vi "MAIN.vi"() -> (2 "digitale waarden reflectiesensor":i32[](array[numeric]))   [LabVIEW 2019]
uses:
  <vilib>/myRIO/Common/Instrument Driver Framework/Utilities/typedefs/Analog Scaling Constants.ctl
  <vilib>/myRIO/Common/Instrument Driver Framework/Utilities/typedefs/Analog Scaling Constants List.ctl
  <vilib>/myRIO/Common/Instrument Driver Framework/myRIO v1.0/AO/typedefs/AO Channels Enum.ctl
  <vilib>/myRIO/Common/Instrument Driver Framework/myRIO v1.0/AO/typedefs/AO Channels List.ctl
  <vilib>/myRIO/Common/Instrument Driver Framework/Utilities/typedefs/Generic FPGA Reference.ctl
  <vilib>/myRIO/Common/Instrument Driver Framework/Utilities/typedefs/myRIO v1.0 Reference.ctl
  <vilib>/myRIO/Common/Instrument Driver Framework/Utilities/typedefs/Hardware Version Enum.ctl
  <vilib>/myRIO/Common/Instrument Driver Framework/Utilities/typedefs/myRIO Generic Hardware Reference.ctl
  <vilib>/myRIO/Instrument Drivers/Onboard IO/AO/typedefs/AO Reference.ctl
  <vilib>/myRIO/Instrument Drivers/Onboard IO/AO/AO.lvlib
  <vilib>/myRIO/Instrument Drivers/Onboard IO/AO/vis/Write.vi
  <vilib>/userDefined/High Color/nirio_resource_hc.ctl
  <vilib>/myRIO/Common/Instrument Driver Framework/myRIO v1.0/AO/vis/myRIO v1.1 Open AO.vi
  <vilib>/myRIO/Instrument Drivers/Onboard IO/AO/vis/myRIO AO Open.xnode
  <vilib>/myRIO/Common/Instrument Driver Framework/Utilities/vis/Is FPGA Ref Available.vi
  <vilib>/myRIO/Express VI/Onboard IO/AO/AO Express VI.xnode
  <vilib>/myRIO/Common/Instrument Driver Framework/myRIO v1.0/AI/typedefs/AI Channels Enum.ctl
  <vilib>/myRIO/Common/Instrument Driver Framework/myRIO v1.0/AI/typedefs/AI Channels List.ctl
  <vilib>/myRIO/Instrument Drivers/Onboard IO/AI/typedefs/AI Reference.ctl
  <vilib>/myRIO/Instrument Drivers/Onboard IO/AI/AI.lvlib
  <vilib>/myRIO/Instrument Drivers/Onboard IO/AI/vis/Read.vi
  <vilib>/myRIO/Common/Instrument Driver Framework/myRIO v1.0/AI/vis/myRIO v1.1 Open AI.vi
  <vilib>/myRIO/Instrument Drivers/Onboard IO/AI/vis/myRIO AI Open.xnode
  <vilib>/myRIO/Express VI/Onboard IO/AI/AI Express VI.xnode
  <vilib>/myRIO/Express VI/Onboard IO/DI/DI Express VI.xnode
  <vilib>/myRIO/Instrument Drivers/Onboard IO/DIO/vis/Read.vi
  <vilib>/myRIO/Instrument Drivers/Onboard IO/DIO/DIO.lvlib
  <vilib>/myRIO/Common/Instrument Driver Framework/myRIO v1.0/DIO/typedefs/DIO Channels Enum.ctl
  <vilib>/myRIO/Common/Instrument Driver Framework/myRIO v1.0/DIO/typedefs/DIO Channels List.ctl
  <vilib>/myRIO/Instrument Drivers/Onboard IO/DIO/typedefs/DIO Reference.ctl
  <vilib>/myRIO/Instrument Drivers/Onboard IO/DIO/vis/myRIO DIO Open.xnode
  <vilib>/myRIO/Common/Instrument Driver Framework/myRIO v1.0/DIO/vis/myRIO v1.1 Open DIO.vi
panel:
  in  "stoppen":bool
  in  "rechts draaien achteruit":bool
  in  "links draaien achteruit":bool
  in  "snelheid":dbl
  in  "rechts draaien":bool
  in  "links draaien":bool
  in  "achterwaarts":bool
  in  "voorwaarts":bool
  out "boolean afstandssensor":bool
  out "High 2":u8[](array[numeric])
  out "Low 2":u8[](array[numeric])
  out "error out":errorcluster
  in  "error in (no error)":errorcluster
  out "Total":u32
  in  "Low":string="–"
  in  "High":string="—"
  out "analoge waarden refelectiesensor":dbl[](array[numeric])
  in  "manuele bedieningknop":bool
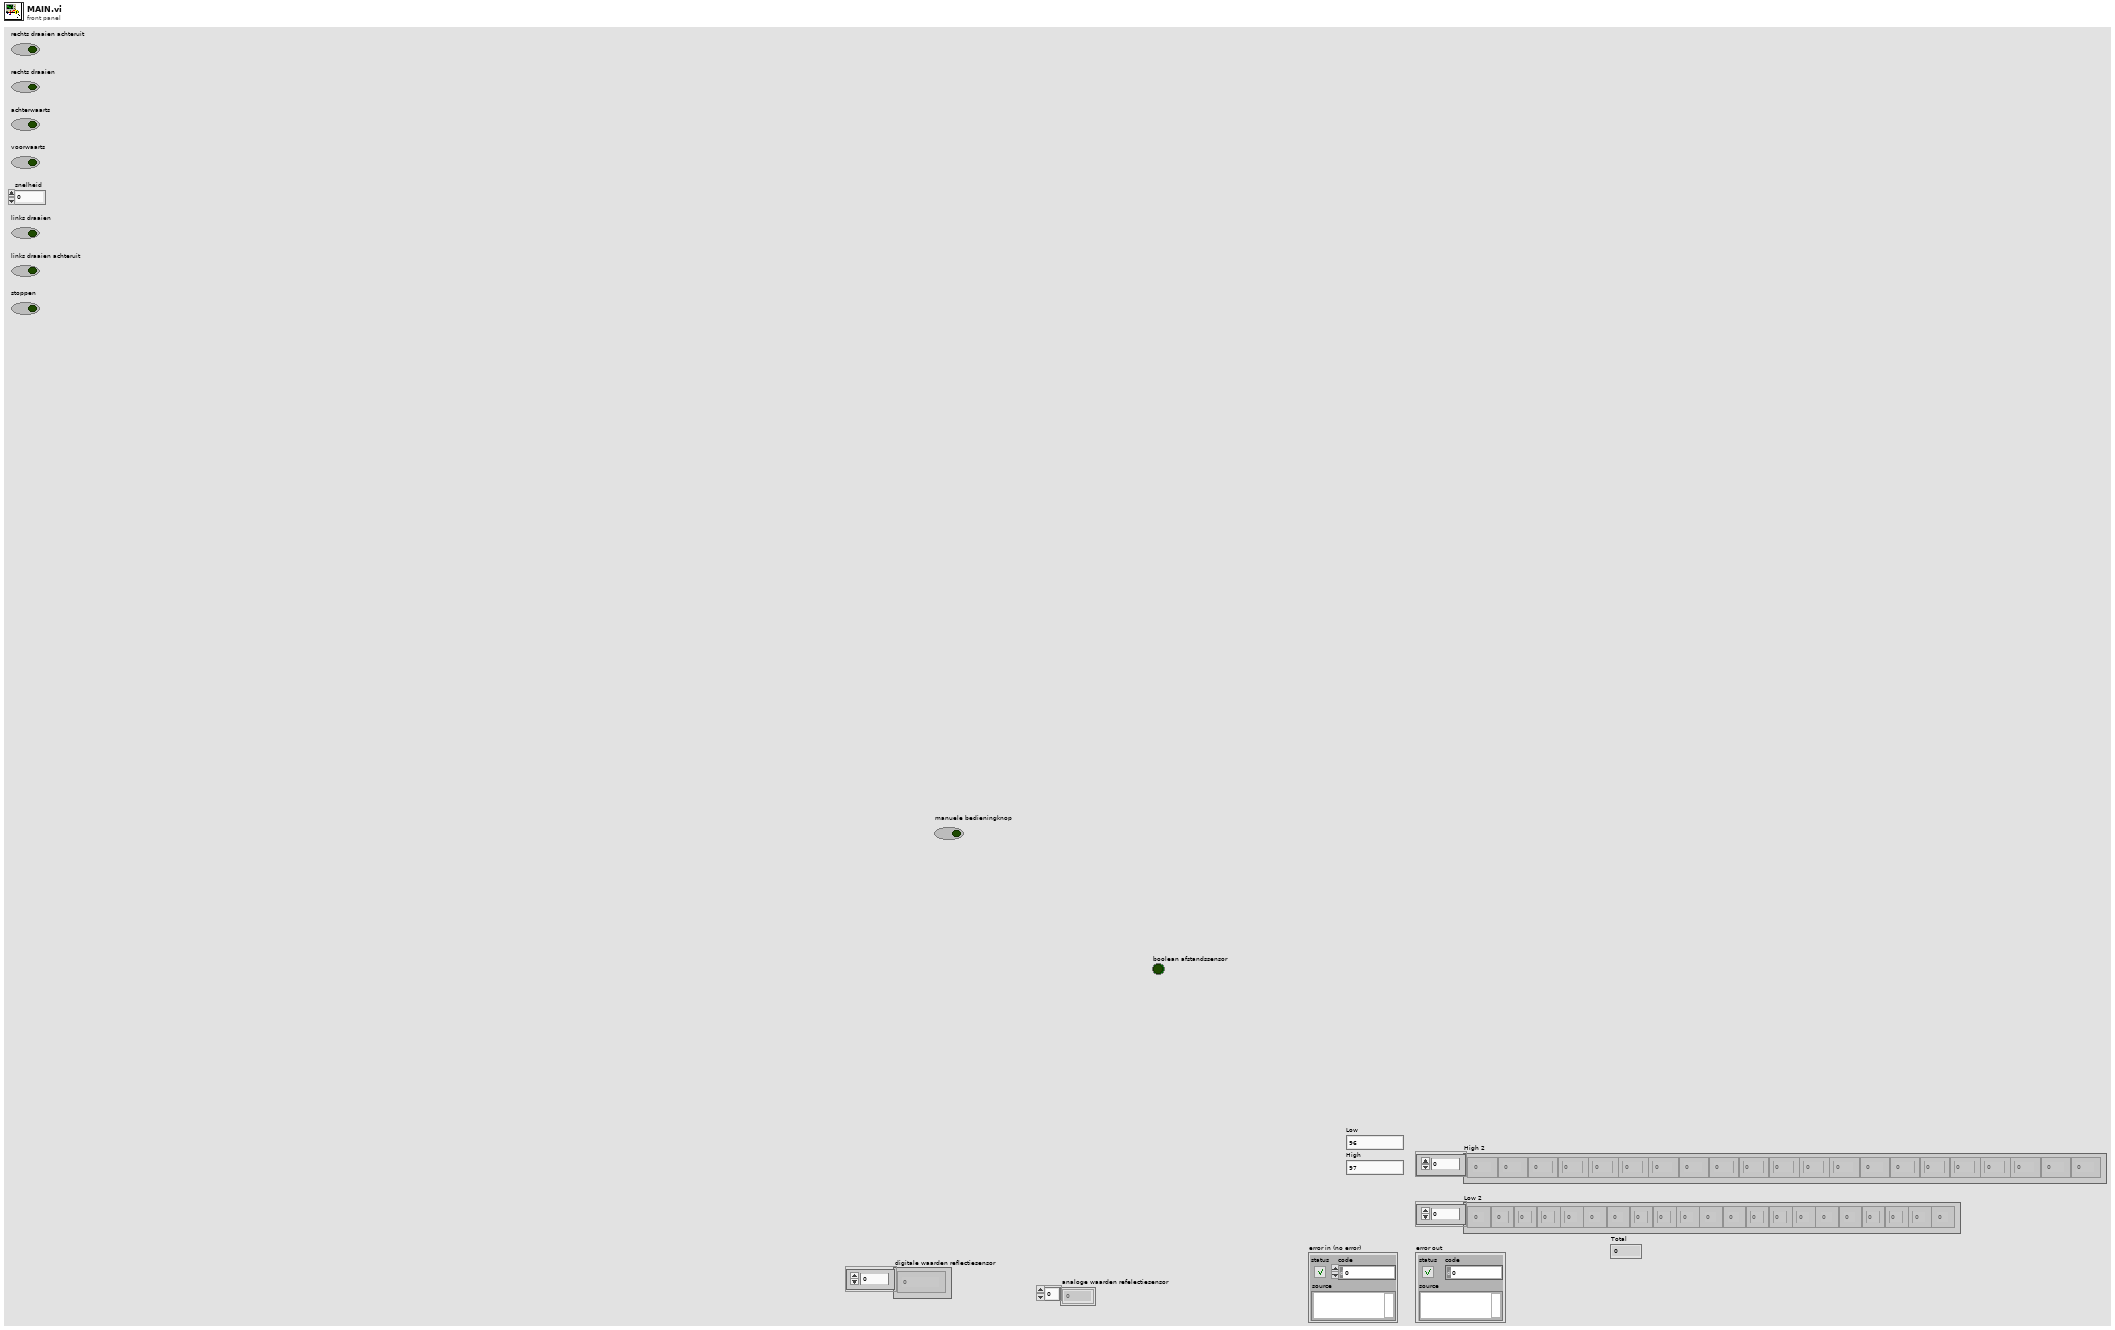
[diagram p1: front panel]
types:
  T1 = typedef "AO.lvlib/AO Reference.ctl" = cluster{"myRIO Reference":T2, "AO Channel List":T6, "AO Scaling Constant List":T8}
  T2 = typedef "myRIO Generic Hardware Reference.ctl" = cluster{"myRIO Model":T3, "myRIO Hardware Reference":T4}
  T3 = typedef "Hardware Version Enum.ctl" = enum16{"Unknown", "myRIO-1900", "myRIO-1950", "roboRIO", "NI ELVIS RIO CM", "ELVIS III"}
  T4 = typedef "myRIO v1.0 Reference.ctl" = cluster{"Generic FPGA Reference":T5, "Allow multiple opens":bool}
  T5 = typedef "Generic FPGA Reference.ctl" = refnum<k20>
  T6 = typedef "AO Channels List.ctl" = T7[]
  T7 = typedef "AO Channels Enum.ctl" = enum16{"Not Connected", "AudioOut/Left", "AudioOut/Right", "C/AO0", "C/AO1", "A/AO0", "A/AO1", "B/AO0", "B/AO1"}
  T8 = typedef "Analog Scaling Constants List.ctl" = T9[]
  T9 = typedef "Analog Scaling Constants.ctl" = cluster{"LSB Weight (Volts)":dbl, "Offset (Volts)":dbl, "Signed?":bool}
  T10 = typedef "nirio_resource_hc.ctl" = tag
  T11 = typedef "AI.lvlib/AI Reference.ctl" = cluster{"myRIO Reference":T2, "AI Channels List":T12, "AI Scaling Constants List":T8}
  T12 = typedef "AI Channels List.ctl" = T13[]
  T13 = typedef "AI Channels Enum.ctl" = enum16{"Not Connected", "AudioIn/Left", "AudioIn/Right", "C/AI0", "C/AI1", "A/AI0", "A/AI1", "A/AI2", "A/AI3", "A/AI4", "A/AI5", "A/AI6", "A/AI7", "B/AI0", "B/AI1", "B/AI2", "B/AI3", "B/AI4", "B/AI5", "B/AI6", "B/AI7", "AI/AI0", "AI/AI1", "AI/AI2", "AI/AI3", "A/AI0 (DIFF)", "A/AI1 (DIFF)", "A/AI2 (DIFF)", "A/AI3 (DIFF)", "B/AI0 (DIFF)", "B/AI1 (DIFF)", "B/AI2 (DIFF)", "B/AI3 (DIFF)"}
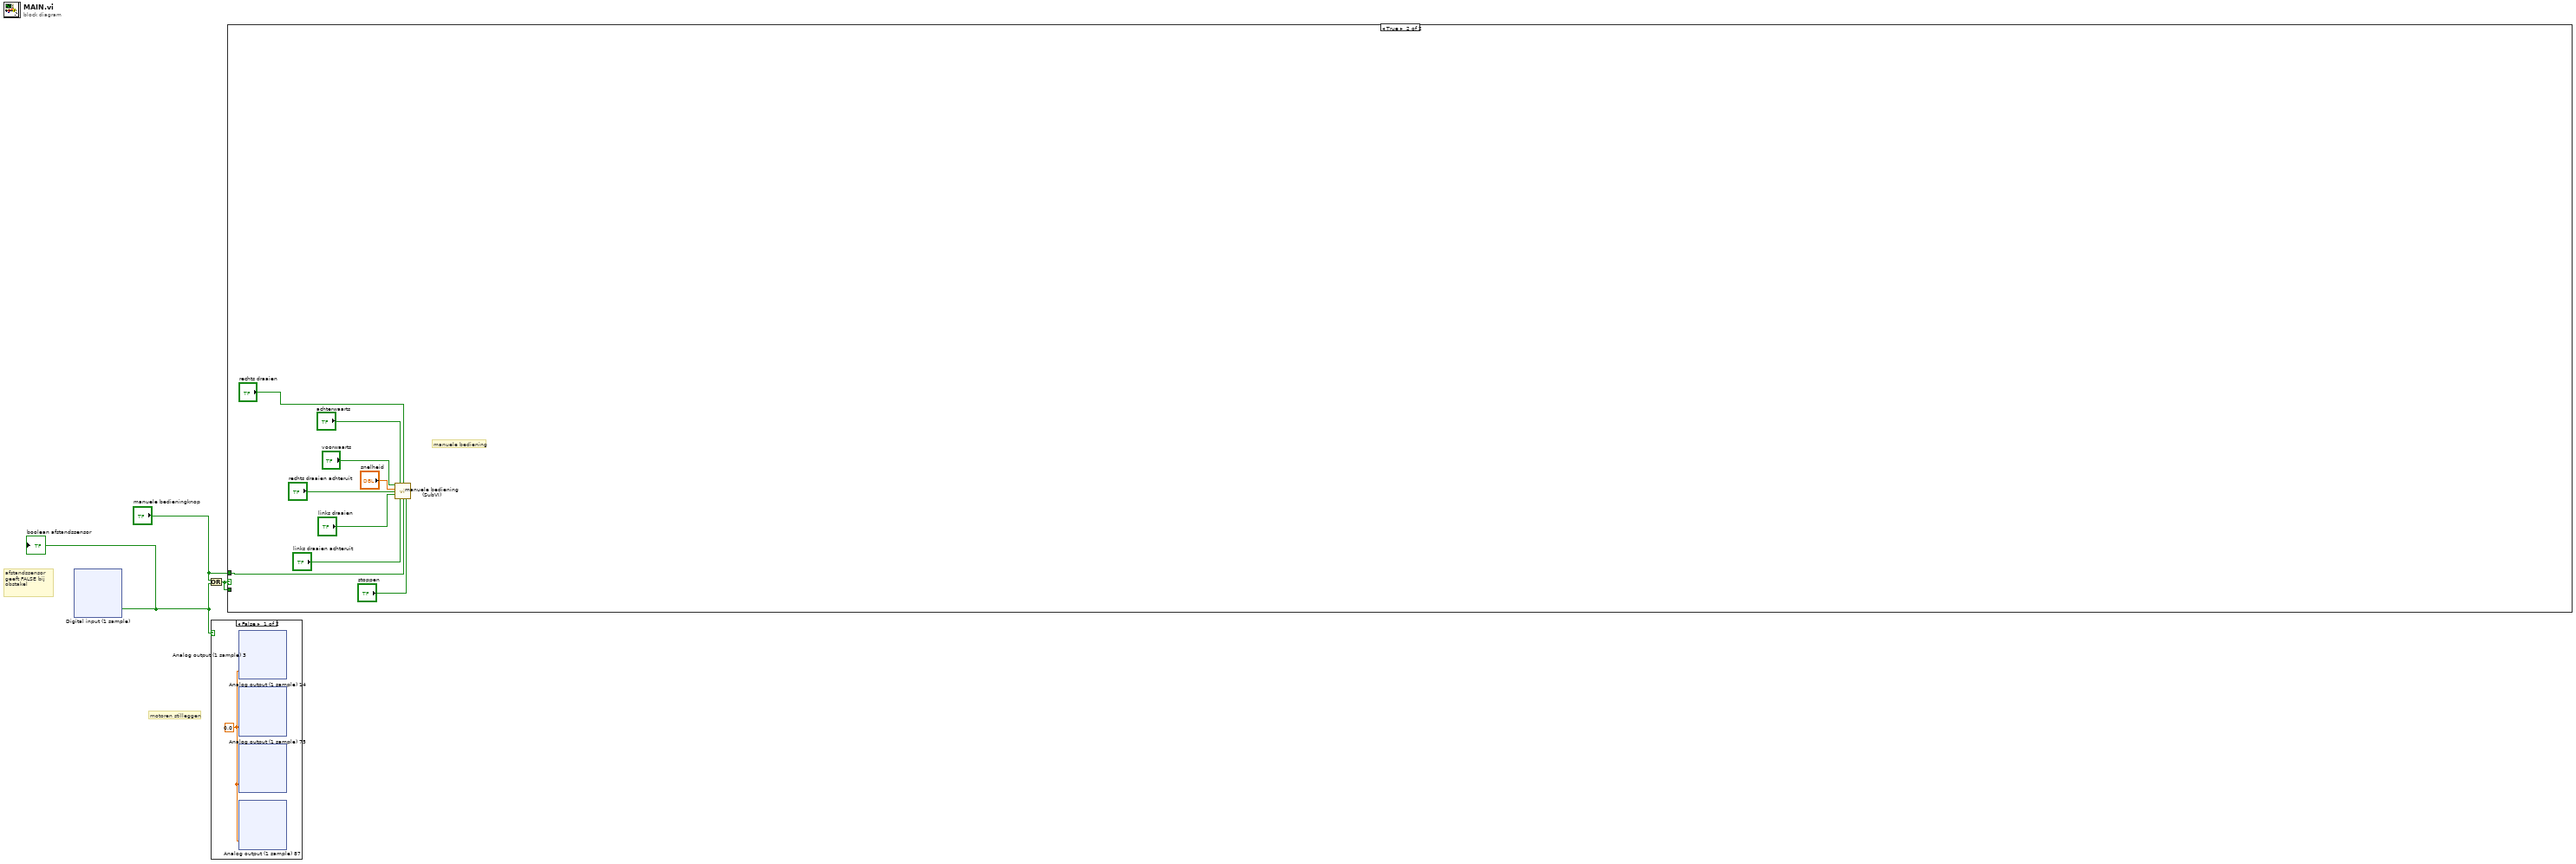
[diagram p0: block diagram]
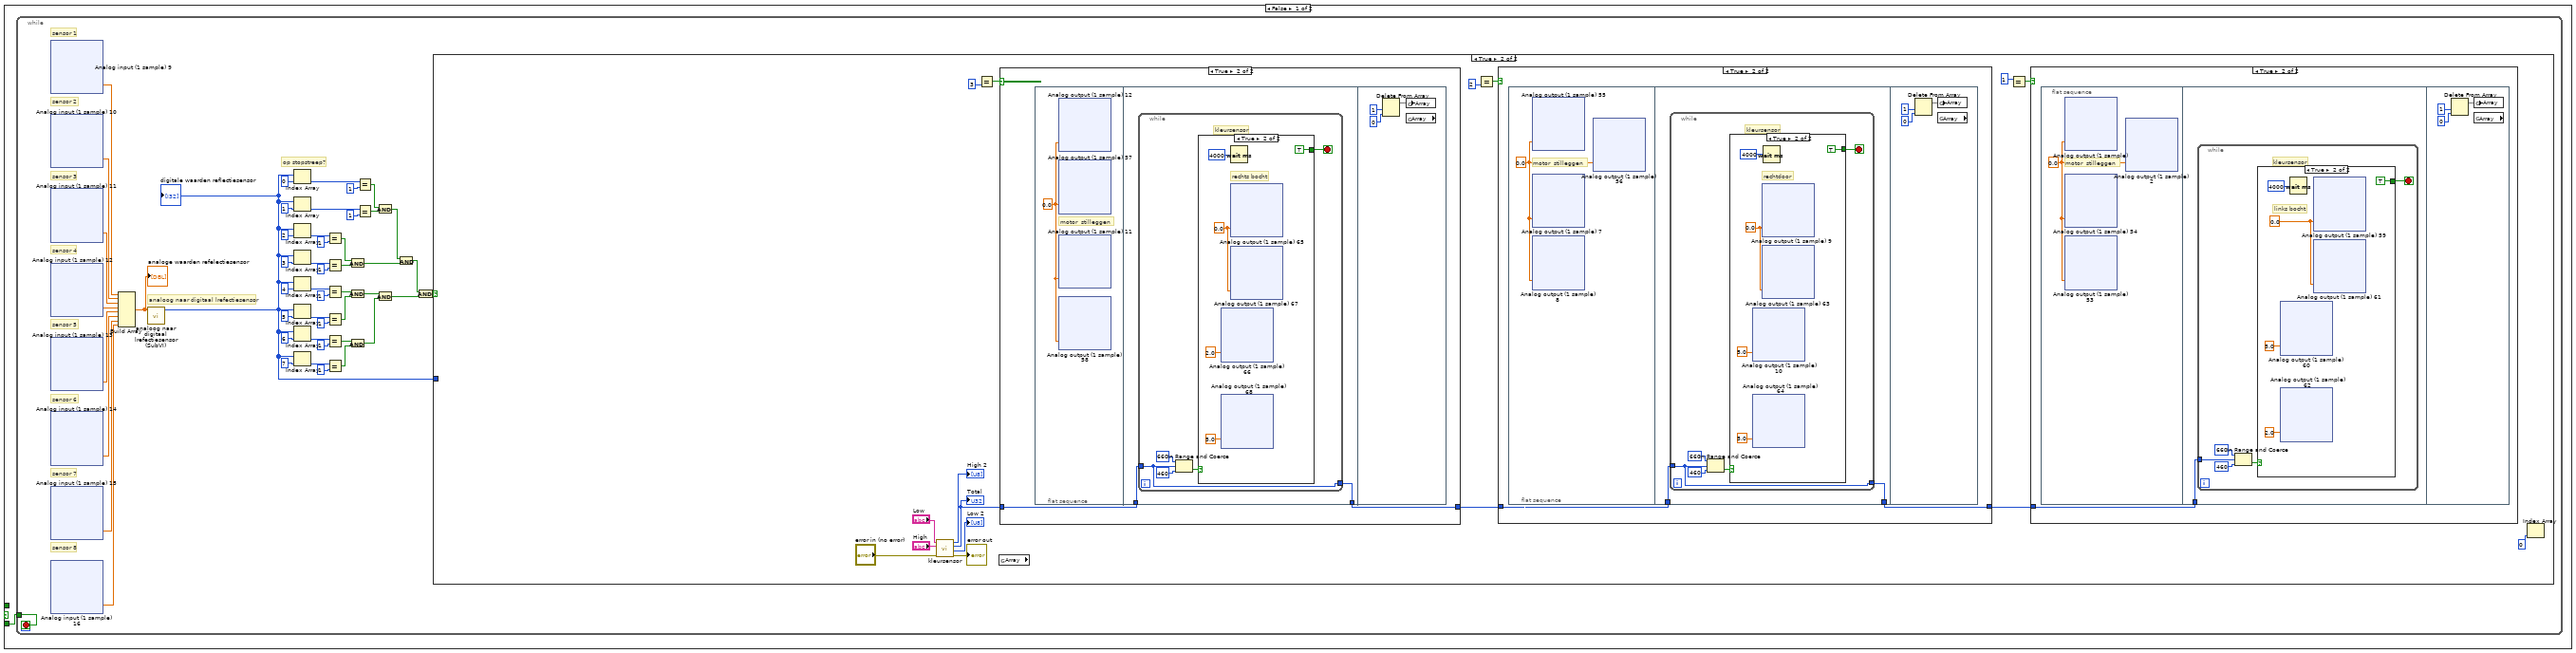
[diagram p3: hidden frame]
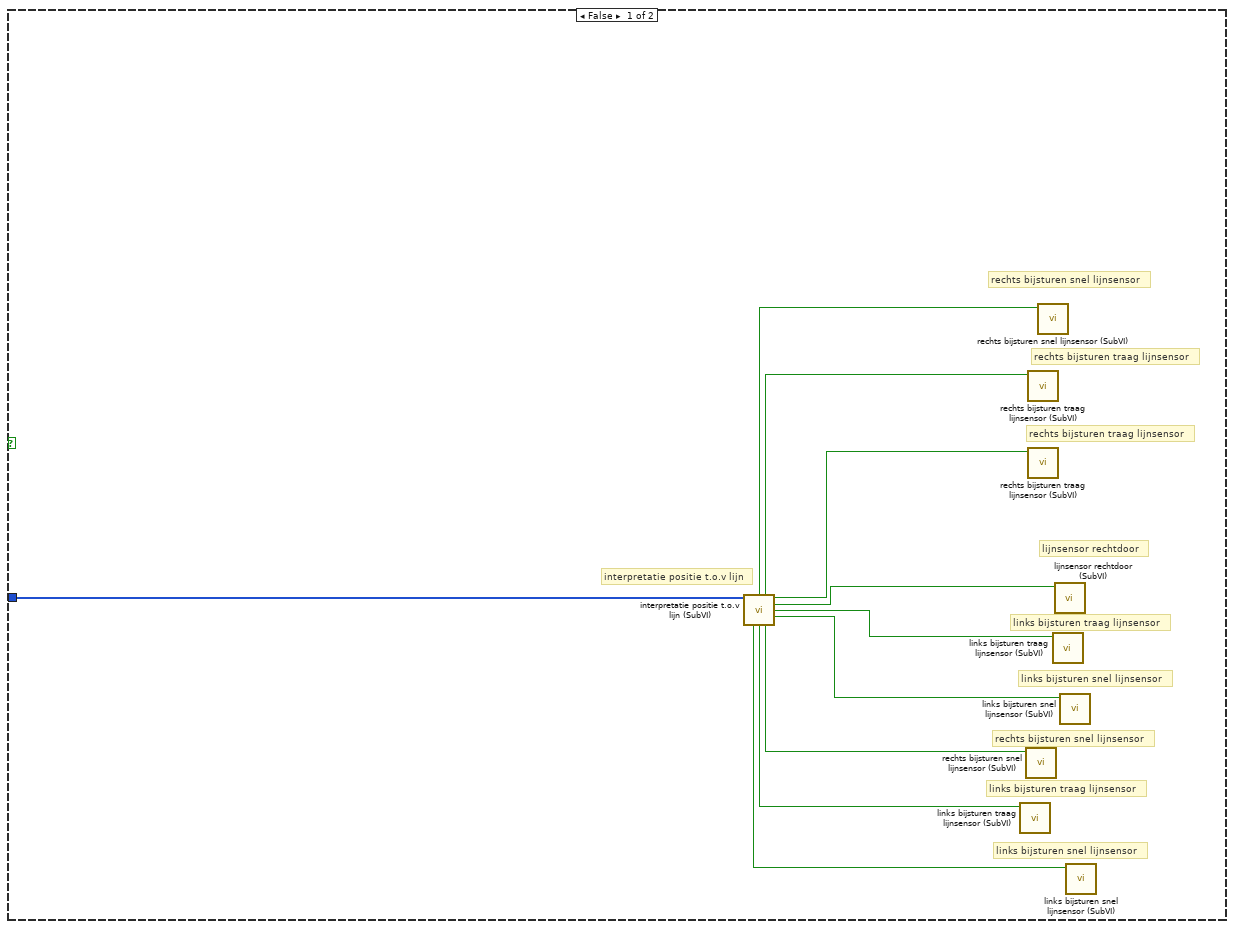
[diagram p4: hidden frame]
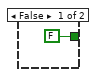
[diagram p6: hidden frame]
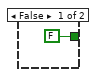
[diagram p8: hidden frame]
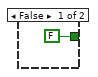
[diagram p10: hidden frame]
diagram:
  # "motoren stilleggen"
  # "afstandssensor \ngeeft FALSE bij obstakel"
  n1 = xnode "Digital input (1 sample)"() -> ("A/DIO1 (Pin 13)"=w1:bool)  [unwired: 1 in, 1 out]
  "boolean afstandssensor" <- w1
  n2 = Or(x="manuele bedieningknop", y=w1) -> (x .or. y?=w3:bool)
  n3 = case shown="False" w1 {
    frame False {
      w4 = 0.0
      n4 = xnode "Analog output (1 sample) 3"("A/AO0 (Pin 2)"=w4) -> ()  [unwired: 1 in, 1 out]
      n5 = xnode "Analog output (1 sample) 14"("A/AO1 (Pin 4)"=w4) -> ()  [unwired: 1 in, 1 out]
      n6 = xnode "Analog output (1 sample) 75"("B/AO0 (Pin 2)"=w4) -> ()  [unwired: 1 in, 1 out]
      n7 = xnode "Analog output (1 sample) 87"("B/AO1 (Pin 4)"=w4) -> ()  [unwired: 1 in, 1 out]
    }
    frame True {
    }
  }
  n8 = case shown="True" w3 {
    tunnel: w3 -> [w153 _]
    tunnel: "manuele bedieningknop" -> [_ w1479]
    frame False {
      n9 = while {
        tunnel: w153 -> [w155]
        stop <- w155 stop-if-true
        # "op stopstreep?"
        # "analoog naar digitaal lrefectiesensor"
        # "sensor 8"
        # "sensor 7"
        # "sensor 6"
        # "sensor 5"
        # "sensor 4"
        # "sensor 3"
        # "sensor 2"
        # "sensor 1"
        n10 = xnode "Analog input (1 sample) 9"() -> ("A/AI3 (Pin 9)"=w164:dbl)  [unwired: 1 in, 1 out]
        n11 = xnode "Analog input (1 sample) 10"() -> ("A/AI2 (Pin 7)"=w163:dbl)  [unwired: 1 in, 1 out]
        n12 = xnode "Analog input (1 sample) 11"() -> ("A/AI1 (Pin 5)"=w162:dbl)  [unwired: 1 in, 1 out]
        n13 = xnode "Analog input (1 sample) 12"() -> ("A/AI0 (Pin 3)"=w161:dbl)  [unwired: 1 in, 1 out]
        n14 = xnode "Analog input (1 sample) 13"() -> ("B/AI3 (Pin 9)"=w160:dbl)  [unwired: 1 in, 1 out]
        n15 = xnode "Analog input (1 sample) 14"() -> ("B/AI2 (Pin 7)"=w159:dbl)  [unwired: 1 in, 1 out]
        n16 = xnode "Analog input (1 sample) 15"() -> ("A/AI1 (Pin 5)"=w158:dbl)  [unwired: 1 in, 1 out]
        n17 = xnode "Analog input (1 sample) 16"() -> ("B/AI0 (Pin 3)"=w157:dbl)  [unwired: 1 in, 1 out]
        n18 = Build Array(w164, w163, w162, w161, w160, w159, w158, w157) -> (w156:dbl[])
        "analoge waarden refelectiesensor" <- w156
        n19 = call "analoog naar digitaal lrefectiesensor (SubVI).vi"("Array in"=w156) -> ("Array out"=w154:i32[])  [unwired: 10 in]
        "digitale waarden reflectiesensor" <- w154
        n20 = Index Array(array=w154, index=0) -> (element=w186:i32)
        n21 = Index Array(array=w154, index=1) -> (element=w165:i32)
        n22 = Index Array(array=w154, index=2) -> (element=w171:i32)
        n23 = Index Array(array=w154, index=3) -> (element=w168:i32)
        n24 = Index Array(array=w154, index=4) -> (element=w174:i32)
        n25 = Index Array(array=w154, index=5) -> (element=w177:i32)
        n26 = Index Array(array=w154, index=6) -> (element=w180:i32)
        n27 = Index Array(array=w154, index=7) -> (element=w183:i32)
        n28 = Equal?(x=w171, y=1) -> (x = y?=w191:bool)
        n29 = Equal?(x=w168, y=1) -> (x = y?=w192:bool)
        n30 = Equal?(x=w174, y=1) -> (x = y?=w193:bool)
        n31 = Equal?(x=w177, y=1) -> (x = y?=w194:bool)
        n32 = Equal?(x=w180, y=1) -> (x = y?=w195:bool)
        n33 = Equal?(x=w183, y=1) -> (x = y?=w196:bool)
        n34 = And(x=w191, y=w192) -> (x .and. y?=w198:bool)
        n35 = And(x=w193, y=w194) -> (x .and. y?=w199:bool)
        n36 = And(x=w195, y=w196) -> (x .and. y?=w200:bool)
        n37 = Equal?(x=w186, y=1) -> (x = y?=w189:bool)
        n38 = Equal?(x=w165, y=1) -> (x = y?=w190:bool)
        n39 = And(x=w189, y=w190) -> (x .and. y?=w197:bool)
        n40 = And(x=w199, y=w200) -> (x .and. y?=w202:bool)
        n41 = And(x=w197, y=w198) -> (x .and. y?=w201:bool)
        n42 = And(x=w201, y=w202) -> (x .and. y?=w203:bool)
        n43 = case shown="True" w203 {
          tunnel: w154 -> [w505 _]
          frame False {
            # "interpretatie positie t.o.v lijn"
            # "rechts bijsturen traag lijnsensor"
            # "rechts bijsturen snel lijnsensor"
            # "links bijsturen snel lijnsensor"
            # "links bijsturen traag lijnsensor"
            # "rechts bijsturen traag lijnsensor"
            # "rechts bijsturen snel lijnsensor"
            # "links bijsturen snel lijnsensor"
            # "links bijsturen traag lijnsensor"
            # "lijnsensor rechtdoor"
            n44 = call "interpretatie positie t.o.v lijn (SubVI).vi"("Array in"=w505) -> ("Boolean 8"=w508:bool, "Boolean 9"=w509:bool, "Boolean"=w500:bool, "Boolean 5"=w504:bool, "Boolean 7"=w507:bool, "Boolean 3"=w502:bool, "Boolean 6"=w506:bool, "Boolean 4"=w503:bool, "Boolean 2"=w501:bool)  [unwired: 6 in]
            n45 = call "links bijsturen traag lijnsensor (SubVI).vi"("Boolean"=w503) -> ()  [unwired: 11 in]
            n46 = call "rechts bijsturen snel lijnsensor (SubVI).vi"("Boolean"=w501) -> ()  [unwired: 11 in]
            n47 = call "rechts bijsturen traag lijnsensor (SubVI).vi"("Boolean"=w509) -> ()  [unwired: 11 in]
            n48 = call "rechts bijsturen traag lijnsensor (SubVI).vi"("Boolean"=w500) -> ()  [unwired: 11 in]
            n49 = call "rechts bijsturen snel lijnsensor (SubVI).vi"("Boolean"=w508) -> ()  [unwired: 11 in]
            n50 = call "links bijsturen traag lijnsensor (SubVI).vi"("Boolean"=w507) -> ()  [unwired: 11 in]
            n51 = call "lijnsensor rechtdoor (SubVI).vi"("Boolean"=w504) -> ()  [unwired: 11 in]
            n52 = call "links bijsturen snel lijnsensor (SubVI).vi"("Boolean"=w502) -> ()  [unwired: 11 in]
            n53 = call "links bijsturen snel lijnsensor (SubVI).vi"("Boolean"=w506) -> ()  [unwired: 11 in]
          }
          frame True {
            n54 = call "kleursensor.vi"("error in (no error)"="error in (no error)", "High in"="High", "Low in"="Low") -> ("error out"=→"error out":errorcluster, "Low out"=→"Low 2":u8[], "Total"=w512:u32, "High out"=→"High 2":u8[])  [unwired: 5 in]
            "Total" <- w512
            n55 = Equal?(y=3) -> (x = y?=w523:bool)  [unwired: 1 in]
            n56 = global read "globalprogram.vi" "Array"() -> ()  [unwired: 1 out]
            n57 = case shown="True" w523 {
              tunnel: w512 -> [w526 w528]
              tunnel: [w526 w527] -> w511
              frame False {
              }
              frame True {
                n58 = flat-sequence {
                  tunnel: w528 -> [w679]
                  tunnel: [w678] -> w527
                  frame #0 {
                    w529 = 0.0
                    # "motor  stilleggen"
                    n59 = xnode "Analog output (1 sample) 12"("A/AO0 (Pin 2)"=w529) -> ()  [unwired: 1 in, 1 out]
                    n60 = xnode "Analog output (1 sample) 57"("A/AO1 (Pin 4)"=w529) -> ()  [unwired: 1 in, 1 out]
                    n61 = xnode "Analog output (1 sample) 11"("B/AO0 (Pin 2)"=w529) -> ()  [unwired: 1 in, 1 out]
                    n62 = xnode "Analog output (1 sample) 58"("B/AO1 (Pin 4)"=w529) -> ()  [unwired: 1 in, 1 out]
                  }
                  frame #1 {
                    n63 = while {
                      tunnel: w679 -> [w680]
                      tunnel: [w680] -> w678
                      stop <- w681 stop-if-true
                      # "kleursensor"
                      n64 = In Range and Coerce(upper limit=660, x=w680, lower limit=460) -> (In Range?=w682:bool)  [unwired: 1 out]
                      n65 = case shown="True" w682 {
                        tunnel: [FALSE TRUE] -> w681
                        frame False {
                        }
                        frame True {
                          w689 = 0.0
                          # "rechts bocht"
                          n66 = xnode "Analog output (1 sample) 66"("A/AO1 (Pin 4)"=2.0) -> ()  [unwired: 1 in, 1 out]
                          n67 = xnode "Analog output (1 sample) 68"("B/AO1 (Pin 4)"=5.0) -> ()  [unwired: 1 in, 1 out]
                          n68 = xnode "Analog output (1 sample) 65"("A/AO0 (Pin 2)"=w689) -> ()  [unwired: 1 in, 1 out]
                          n69 = xnode "Analog output (1 sample) 67"("B/AO0 (Pin 2)"=w689) -> ()  [unwired: 1 in, 1 out]
                          n70 = Wait (ms)(milliseconds to wait=u32 4000) -> ()  [unwired: 1 out]
                        }
                      }
                    }
                  }
                  frame #2 {
                    n71 = Delete From Array(length=1, index=0) -> (array with subset deleted=w841)  [unwired: 1 in, 1 out]
                    n72 = global write "globalprogram.vi" "Array"(w841) -> ()
                    n73 = global read "globalprogram.vi" "Array"() -> ()  [unwired: 1 out]
                  }
                }
              }
            }
            n74 = Equal?(y=2) -> (x = y?=w524:bool)  [unwired: 1 in]
            n75 = case shown="True" w524 {
              tunnel: w511 -> [w1155 w1157]
              tunnel: [w1155 w1156] -> w510
              frame False {
              }
              frame True {
                n76 = flat-sequence {
                  tunnel: w1157 -> [w1308]
                  tunnel: [w1307] -> w1156
                  frame #0 {
                    w1158 = 0.0
                    # "motor  stilleggen"
                    n77 = xnode "Analog output (1 sample) 55"("A/AO1 (Pin 4)"=w1158) -> ()  [unwired: 1 in, 1 out]
                    n78 = xnode "Analog output (1 sample) 7"("B/AO0 (Pin 2)"=w1158) -> ()  [unwired: 1 in, 1 out]
                    n79 = xnode "Analog output (1 sample) 8"("A/AO0 (Pin 2)"=w1158) -> ()  [unwired: 1 in, 1 out]
                    n80 = xnode "Analog output (1 sample) 56"("B/AO1 (Pin 4)"=w1158) -> ()  [unwired: 1 in, 1 out]
                  }
                  frame #1 {
                    n81 = while {
                      tunnel: w1308 -> [w1309]
                      tunnel: [w1309] -> w1307
                      stop <- w1310 stop-if-true
                      # "kleursensor"
                      n82 = In Range and Coerce(upper limit=660, x=w1309, lower limit=460) -> (In Range?=w1311:bool)  [unwired: 1 out]
                      n83 = case shown="True" w1311 {
                        tunnel: [FALSE TRUE] -> w1310
                        frame False {
                        }
                        frame True {
                          w1318 = 0.0
                          # "rechtdoor"
                          n84 = xnode "Analog output (1 sample) 10"("A/AO1 (Pin 4)"=5.0) -> ()  [unwired: 1 in, 1 out]
                          n85 = xnode "Analog output (1 sample) 64"("B/AO1 (Pin 4)"=5.0) -> ()  [unwired: 1 in, 1 out]
                          n86 = xnode "Analog output (1 sample) 9"("A/AO0 (Pin 2)"=w1318) -> ()  [unwired: 1 in, 1 out]
                          n87 = xnode "Analog output (1 sample) 63"("B/AO0 (Pin 2)"=w1318) -> ()  [unwired: 1 in, 1 out]
                          n88 = Wait (ms)(milliseconds to wait=u32 4000) -> ()  [unwired: 1 out]
                        }
                      }
                    }
                  }
                  frame #2 {
                    n89 = Delete From Array(length=1, index=0) -> (array with subset deleted=w1470)  [unwired: 1 in, 1 out]
                    n90 = global write "globalprogram.vi" "Array"(w1470) -> ()
                    n91 = global read "globalprogram.vi" "Array"() -> ()  [unwired: 1 out]
                  }
                }
              }
            }
            n92 = Equal?(x=1) -> (x = y?=w525:bool)  [unwired: 1 in]
            n93 = case shown="True" w525 {
              tunnel: w510 -> [_ w842]
              frame False {
              }
              frame True {
                n94 = flat-sequence {
                  tunnel: w842 -> [w992]
                  frame #0 {
                    w843 = 0.0
                    # "motor  stilleggen"
                    n95 = xnode "Analog output (1 sample)"("A/AO1 (Pin 4)"=w843) -> ()  [unwired: 1 in, 1 out]
                    n96 = xnode "Analog output (1 sample) 54"("B/AO1 (Pin 4)"=w843) -> ()  [unwired: 1 in, 1 out]
                    n97 = xnode "Analog output (1 sample) 53"("A/AO0 (Pin 2)"=w843) -> ()  [unwired: 1 in, 1 out]
                    n98 = xnode "Analog output (1 sample) 2"("B/AO0 (Pin 2)"=w843) -> ()  [unwired: 1 in, 1 out]
                  }
                  frame #1 {
                    n99 = while {
                      tunnel: w992 -> [w993]
                      stop <- w994 stop-if-true
                      # "kleursensor"
                      n100 = In Range and Coerce(upper limit=660, x=w993, lower limit=460) -> (In Range?=w995:bool)  [unwired: 1 out]
                      n101 = case shown="True" w995 {
                        tunnel: [FALSE TRUE] -> w994
                        frame False {
                        }
                        frame True {
                          w1001 = 0.0
                          # "links bocht"
                          n102 = xnode "Analog output (1 sample) 60"("A/AO1 (Pin 4)"=5.0) -> ()  [unwired: 1 in, 1 out]
                          n103 = xnode "Analog output (1 sample) 62"("B/AO1 (Pin 4)"=2.0) -> ()  [unwired: 1 in, 1 out]
                          n104 = Wait (ms)(milliseconds to wait=u32 4000) -> ()  [unwired: 1 out]
                          n105 = xnode "Analog output (1 sample) 59"("A/AO0 (Pin 2)"=w1001) -> ()  [unwired: 1 in, 1 out]
                          n106 = xnode "Analog output (1 sample) 61"("B/AO0 (Pin 2)"=w1001) -> ()  [unwired: 1 in, 1 out]
                        }
                      }
                    }
                  }
                  frame #2 {
                    n107 = Delete From Array(length=1, index=0) -> (array with subset deleted=w1154)  [unwired: 1 in, 1 out]
                    n108 = global write "globalprogram.vi" "Array"(w1154) -> ()
                    n109 = global read "globalprogram.vi" "Array"() -> ()  [unwired: 1 out]
                  }
                }
              }
            }
            n110 = Index Array(index=0) -> ()  [unwired: 1 in, 1 out]
          }
        }
      }
    }
    frame True {
      # "manuele bediening"
      n111 = call "manuele bediening (SubVI).vi"("voorwaarts"="voorwaarts", "achterwaarts"="achterwaarts", "rechts draaien"="rechts draaien", "snelheid"="snelheid", "rechts draaien achteruit"="rechts draaien achteruit", "links draaien"="links draaien", "links draaien achteruit"="links draaien achteruit", "Boolean manueel"=w1479, "stoppen"="stoppen") -> ()  [unwired: 7 in]
    }
  }
